vi "ws Spartan Config.vi"(10 "default value (\"\")":string, 11 "config key (\"\")":string) -> (2 "found key?":bool, 3 "config value":string, 5 "CONFIG":T1)   [LabVIEW 2011]
uses:
  <vilib>/addons/internet/utils/keyedarr.llb/Keyed Array.ctl
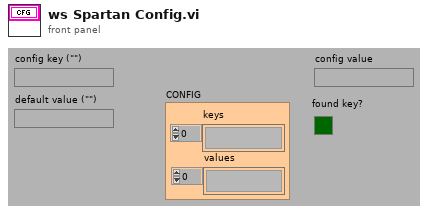
[diagram p1: front panel]
types:
  T1 = typedef "Keyed Array.ctl" = cluster{"keys":string[], "values":string[]}
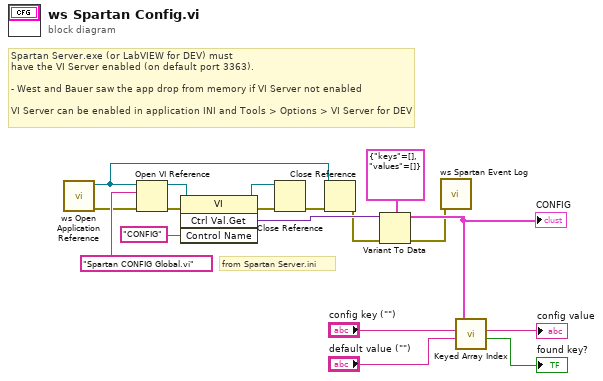
[diagram p0: block diagram]
diagram:
  # "Spartan Server.exe (or LabVIEW for DEV) must\nhave the VI Server enabled (on default port 3363).\n\n- West and Bauer saw the app drop from memory if VI Server not enabled\n\nVI Server can be enabled in application INI and Tools > Options > VI Server for DEV"
  # "from Spartan Server.ini"
  n1 = call "ws Open Application Reference.vi"() -> ("error out"=w3:errorcluster, "application reference"=w2:refnum<vi>)  [unwired: 10 in]
  n2 = Open VI Reference(application reference (local)=w2, vi path="Spartan CONFIG Global.vi", error in (no error)=w3) -> (vi reference=w6:refnum<vi>, error out=w7:errorcluster)  [unwired: 3 in]
  n3 = invoke class="VI" method="Ctrl Val.Get"(reference=w6, error in=w7, "Control Name"="CONFIG") -> (reference out=w10:refnum<vi>, error out=w11:errorcluster, "Get Control Value Variant"=w12:variant)  [unwired: 1 in, 1 out]
  n4 = Close Reference(reference=w10, error in (no error)=w11) -> (error out=w5:errorcluster)
  n5 = Close Reference(reference=w2, error in (no error)=w5) -> (error out=w4:errorcluster)
  n6 = Variant To Data(error in=w4, type=T1 {"keys"=[], "values"=[]} ("CONFIG"), Variant=w12) -> (data=w18:T1, error out=w1:errorcluster)
  "CONFIG" <- w18
  n7 = call "ws Spartan Event Log.vi"("error in (no error)"=w1) -> ()  [unwired: 7 in, 1 out]
  n8 = call <vilib>:"Keyed Array Index.vi"("default value"="default value (\"\")", "key"="config key (\"\")", "array in"=w18) -> ("valid key"=→"found key?":bool, "value"=→"config value":string)  [unwired: 1 in, 2 out]
